vi "ep_Short Impedance (1ch).vi"(0 "fundamental voltage vectors":cdb[](array[numeric]), 1 "restart (F)":bool, 5 "voltage range*sensitivity":dbl, 7 "fundamental current vectors":cdb[](array[numeric]), 9 "current range*sensitivity":dbl) -> (4 "short impedance":cdb)   [LabVIEW 2011, in "NI_EP_Power Quality.lvlib"]
uses:
  <vilib>/addons/Electrical Power/PQ/NI_EP_Power Quality.lvlib
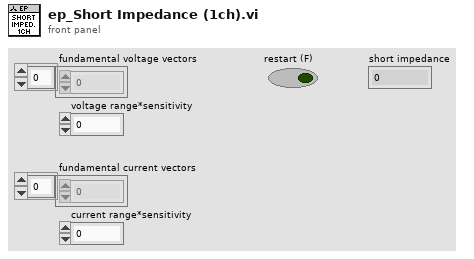
[diagram p1: front panel]
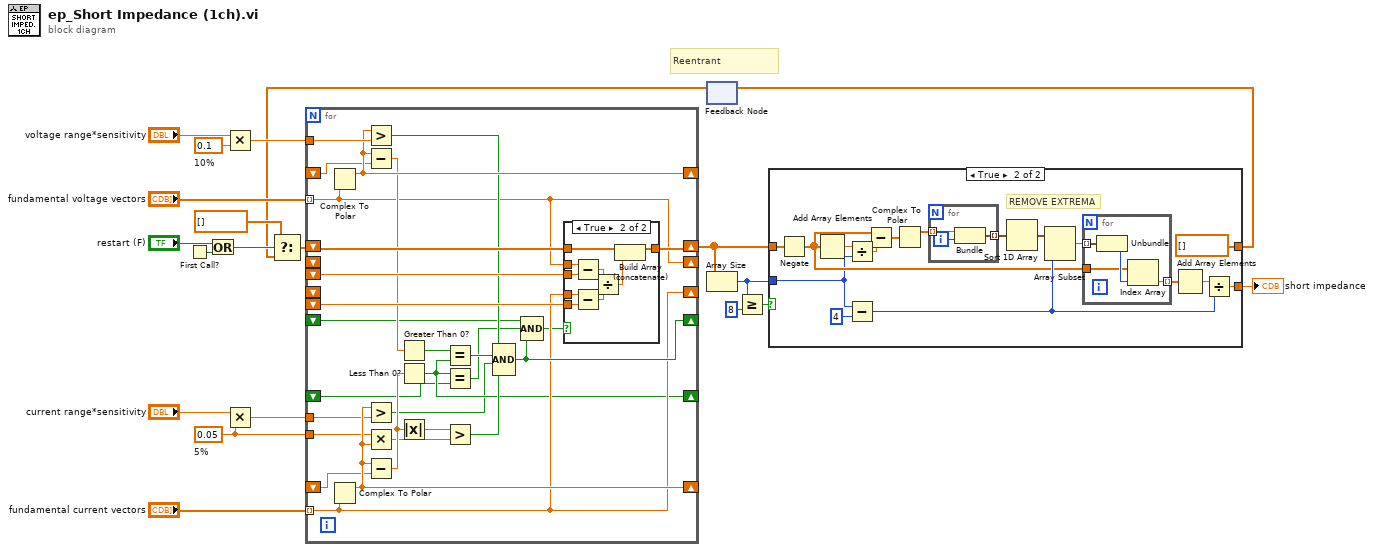
[diagram p0: block diagram]
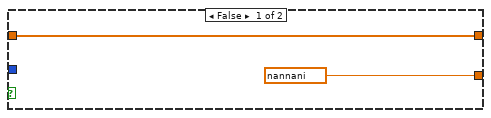
[diagram p2: hidden frame]
diagram:
  w20 = 0.1  # 10%
  w13 = 0.05  # 5%
  # "Reentrant"
  n1 = First Call?() -> (First Call?: T/F=w6:bool)
  n2 = Or(x="restart (F)", y=w6) -> (x .or. y?=w4:bool)
  n3 = Multiply(x="voltage range*sensitivity", y=w20) -> (x*y=w19:dbl)
  n4 = Multiply(x="current range*sensitivity", y=w13) -> (x*y=w18:dbl)
  n5 = feedback #1() -> (w1:cdb[])  [unwired: 1 in]
  n6 = Select(t=cdb[] [] ("Array 2"), s=w4, f=w1) -> (s? t:f=w2:cdb[])
  n7 = for {
    shift-right: [w48] -> w15
    shift-left: w2 -> [w47]
    tunnel: "fundamental voltage vectors" -> [w27] mode=indexing
    tunnel: "fundamental current vectors" -> [w28] mode=indexing
    shift-right: [w30] -> _
    shift-left: _ -> [w24]
    shift-right: [w27] -> _
    shift-left: _ -> [_]
    shift-left: _ -> [w45]
    shift-right: [w28] -> _
    shift-left: _ -> [_]
    shift-left: _ -> [w46]
    tunnel: w19 -> [w44]
    shift-right: [w43] -> _
    shift-left: _ -> [w29]
    shift-right: [w39] -> _
    shift-left: _ -> [w38]
    tunnel: w18 -> [w36]
    tunnel: w13 -> [w37]
    shift-right: [w26] -> _
    shift-left: _ -> [w22]
    n8 = Complex To Polar(r * e^(i*theta)=w27) -> (r=w43:dbl)  [unwired: 1 out]
    n9 = Complex To Polar(r * e^(i*theta)=w28) -> (r=w39:dbl)  [unwired: 1 out]
    n10 = Greater?(x=w43, y=w44) -> (0:w31:bool)
    n11 = Subtract ("dU")(x=w43, y=w29) -> (x-y=w42:dbl)
    n12 = Greater?(x=w39, y=w36) -> (0:w25:bool)
    n13 = Multiply(x=w37, y=w39) -> (x*y=w35:dbl)
    n14 = Subtract ("dU")(x=w39, y=w38) -> (x-y=w40:dbl)
    n15 = Greater Than 0?(x=w42) -> (x > 0?=w33:bool)
    n16 = Less Than 0?(x=w40) -> (x < 0?=w26:bool)
    n17 = Absolute Value(x=w40) -> (abs(x)=w41:dbl)
    n18 = Equal?(x=w33, y=w26) -> (x = y?=w32:bool)
    n19 = Equal?(x=w26, y=w22) -> (x = y?=w23:bool)
    n20 = Greater?(x=w41, y=w35) -> (0:w34:bool)
    n21 = Compound Arithmetic op=AND(w31, w32, w25, w34) -> (w30:bool)
    n22 = Compound Arithmetic op=AND(w24, w23, w30) -> (w21:bool)
    n23 = case shown="True" w21 {
      tunnel: w27 -> [_ w56]
      tunnel: [w49 w58] -> w48
      tunnel: w47 -> [w49 w57]
      tunnel: w28 -> [_ w54]
      tunnel: w45 -> [_ w55]
      tunnel: w46 -> [_ w53]
      frame False {
      }
      frame True {
        n24 = Subtract(x=w56, y=w55) -> (x-y=w52:cdb)
        n25 = Subtract(x=w54, y=w53) -> (x-y=w51:cdb)
        n26 = Divide(x=w52, y=w51) -> (x/y=w50:cdb)
        n27 = Build Array (concatenate)(w57, w50) -> (w58:cdb[])
      }
    }
  }
  n28 = Array Size(array=w15) -> (size(s)=w12:i32)
  n29 = Greater Or Equal?(x=w12, y=8) -> (x >= y?=w16:bool)
  n30 = case shown="True" w16 {
    tunnel: w15 -> [w60 w75]
    tunnel: w12 -> [_ w61]
    tunnel: [w60 cdb[] [] ("Array 2")] -> w14
    tunnel: [cdb nan+nani ("mean") w63] -> w7
    frame False {
    }
    frame True {
      # "REMOVE EXTREMA"
      n31 = Negate(x=w75) -> (-x=w62:cdb[])
      n32 = Add Array Elements(numeric array=w62) -> (sum=w64:cdb)
      n33 = Divide(x=w64, y=w61) -> (x/y=w74:cdb)
      n34 = Subtract(x=w61, y=4) -> (x-y=w72:i32)
      n35 = Subtract(x=w62, y=w74) -> (x-y=w65:cdb[])
      n36 = Complex To Polar(r * e^(i*theta)=w65) -> (r=w66:dbl[])  [unwired: 1 out]
      n37 = for {
        tunnel: w66 -> [w83] mode=indexing
        tunnel: [w81] -> w67 mode=indexing
        i -> [w82]
        n38 = Bundle(w83, w82) -> (w81:cluster{dbl, i32})  [unwired: 1 in]
      }
      n39 = Sort 1D Array(array=w67) -> (sorted array=w73:cluster{dbl, i32}[])
      n40 = Array Subset(array=w73, length=w72) -> (w69:cluster{dbl, i32}[])  [unwired: 1 in]
      n41 = for {
        tunnel: w69 -> [w80] mode=indexing
        tunnel: w62 -> [w78]
        tunnel: [w77] -> w70 mode=indexing
        n42 = Unbundle(w80) -> (w79:i32)  [unwired: 1 out]
        n43 = Index Array(array=w78, index=w79) -> (element=w77:cdb)
      }
      n44 = Add Array Elements(numeric array=w70) -> (sum=w71:cdb)
      n45 = Divide(x=w71, y=w72) -> (x/y=w63:cdb)
    }
  }
  "short impedance" <- w7
  n46 = feedback-in #1(w14) -> ()
